vi "Configure Input Settings.vi"(0 "VISA resource name":refnum<visa-resource-name>, 1 "Channel (1)":u16(ring)=1 items=["All Channels (0)", "1", "2", "3", "4", "5", "6", "7", "8", "9", "10", "11", "12", "13", "14", "15", "16", "A (Control Input)"], 2 "Scan Dwell Time (10)":dbl=10.0 min=1.0 max=200.0 step=1.0, 3 "Change Pause Time (3)":dbl=3.0 min=3.0 max=200.0 step=1.0, 4 "Curve Number (0)":i32 min=0 max=59 step=1, 5 "error in (no error)":errorcluster, 6 "Enable Channel (T: Enable)":bool=TRUE, 7 "Enable Filter (F: Off)":bool, 8 "Temperature Coefficient (1: Negative)":u16(ring)=1 items=["Negative"=1, "Positive"=2], 9 "Settle Time (10 sec)":i32=10 min=1 max=200 step=1, 10 "Input Name":string, 11 "Window (40% FS)":i32=40 min=1 max=80 step=1) -> (14 "VISA resource name out":refnum<visa-resource-name>, 19 "error out":errorcluster)   [LabVIEW 2018, in "Lake Shore 372.lvlib"]
doc: "Configures the 372 input setup. The VI sets input channel parameters for the commands <B>INSET</B>, <B>INNAME</B>, and <B>FILTER</B>. Please refer to Model 372 for further explanation.\n\nNotes: \nAt least one measurement input channel must be enables. If all are configured to disables, channel 1 will change to enabled.\nWhen the filter is on and the settle time is zero, the instrument continues to calculate the filtered reading, despite the unfiltered readings being displayed. This feature allows the user to quickly toggle between 0 s and the desired settle time to observe the filtering effects on the reading. See Model 372 manual section 4.4.7 for more information."
uses:
  Lake Shore 372.lvlib
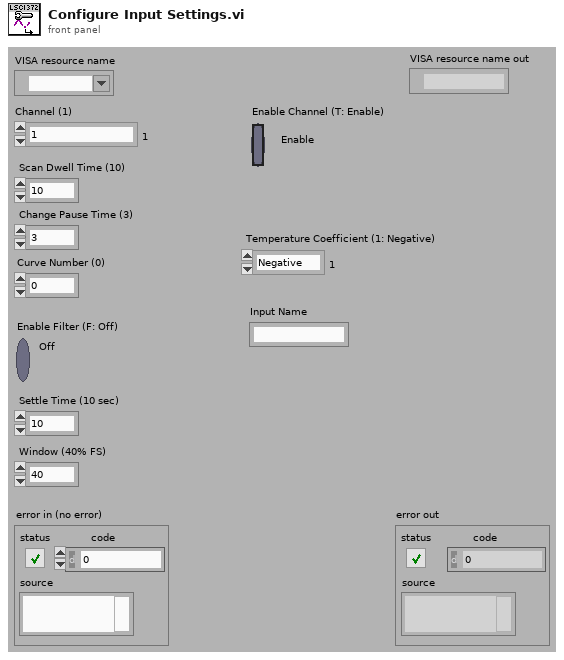
[diagram p1: front panel]
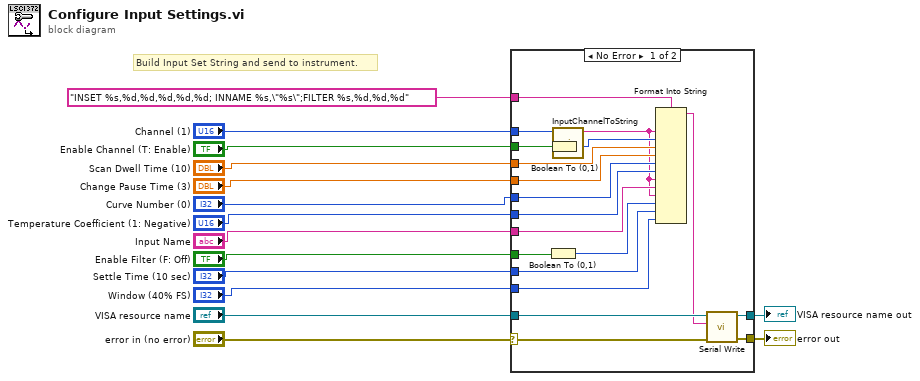
[diagram p0: block diagram]
diagram:
  # "Build Input Set String and send to instrument."
  n1 = case shown="No Error" "error in (no error)" {
    selector: "error in (no error)" -> [w16 w35]
    tunnel: "INSET %s,%d,%d,%d,%d,%d; INNAME %s,\"%s\";FILTER %s,%d,%d,%d" -> [w34 _]
    tunnel: "VISA resource name" -> [w32 w36]
    tunnel: [w31 w35] -> w13
    tunnel: [w30 w36] -> w12
    tunnel: "Enable Channel (T: Enable)" -> [w28 _]
    tunnel: "Scan Dwell Time (10)" -> [w27 _]
    tunnel: "Change Pause Time (3)" -> [w26 _]
    tunnel: "Curve Number (0)" -> [w25 _]
    tunnel: "Temperature Coefficient (1: Negative)" -> [w24 _]
    tunnel: "Channel (1)" -> [w23 _]
    tunnel: "Enable Filter (F: Off)" -> [w22 _]
    tunnel: "Settle Time (10 sec)" -> [w21 _]
    tunnel: "Window (40% FS)" -> [w20 _]
    tunnel: "Input Name" -> [w18 _]
    frame No Error {
      n2 = Boolean To (0,1)(Boolean=w22) -> (0, 1=w19:i16)
      n3 = Boolean To (0,1)(Boolean=w28) -> (0, 1=w33:i16)
      n4 = call "InputChannelToString.vi"("Channel (1)"=w23) -> ("Channel Str"=w17:string)  [unwired: 10 in]
      n5 = Format Into String(format string=w34, w17, w33, w27, w26, w25, w24, w17, w18, w17, w19, w21, w20) -> (resulting string=w29:string)  [unwired: 2 in, 1 out]
      n6 = call "Serial Write.vi"("error in (no error)"=w16, "Write Buffer (\"\")"=w29, "VISA resource name"=w32) -> ("error out"=w31:errorcluster, "VISA resource name out"=w30:refnum<visa-resource-name>)  [unwired: 6 in, 1 out]
    }
    frame Error {
    }
  }
  "error out" <- w13
  "VISA resource name out" <- w12
